vi "AutoVisionShoot.vi"(6 "Drive Params":T1={"Omni"=TRUE, "Low Gear"=TRUE}, 9 "Reset?":bool, 11 "Array":dbl[](array[numeric]) format="%0.3f") -> (3 "isFinished":bool)   [LabVIEW 2013]
uses:
  Shooter/Shooter Command.ctl
  Robot Global Data.vi
  Shooter/Shooter Manual Control.ctl
  Drivetrain/DT Mode.ctl
  Drivetrain/Drivetrain Control.ctl
  AutoDriveParams.ctl
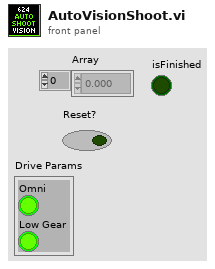
[diagram p1: front panel]
types:
  T1 = typedef "AutoDriveParams.ctl" = cluster{"Omni":bool, "Low Gear":bool}
  T2 = typedef "DT Mode.ctl" = enum16{"Manual", "Ball Steer", "Gyro Steer", "Goal Steer", "Catch Steer", "Selfcatch", "Ball Drive", "Distance Drive"}
  T3 = typedef "Drivetrain Control.ctl" = cluster{"axis 1 (x)":dbl, "axis 2 (y)":dbl, "Mode":T2, "heading target":dbl, "steer axis":dbl, "omni?":bool, "Low Gear?":bool, "distance target":cluster{"x":dbl, "y":dbl}, "PID Params":cluster{"X Dist":cluster{"PID gains":cluster{"proportional gain (Kc)":dbl, "integral time (Ti, min)":dbl, "derivative time (Td, min)":dbl}, "output range":cluster{"output high":dbl, "output low":dbl}}, "Y Dist":cluster{"PID gains":cluster{"proportional gain (Kc)":dbl, "integral time (Ti, min)":dbl, "derivative time (Td, min)":dbl}, "output range":cluster{"output high":dbl, "output low":dbl}}}, "Coast":bool}
  T4 = typedef "Shooter Manual Control.ctl" = cluster{"Command":T5, "Offset":dbl, "Trigger":bool, "Add":bool, "Release":bool, "Reset":bool, "Target Pressure":dbl, "Punch":bool, "AutoPunch":bool}
  T5 = typedef "Shooter Command.ctl" = enum16{"None", "Warmup", "Shoot", "Line Shoot"}
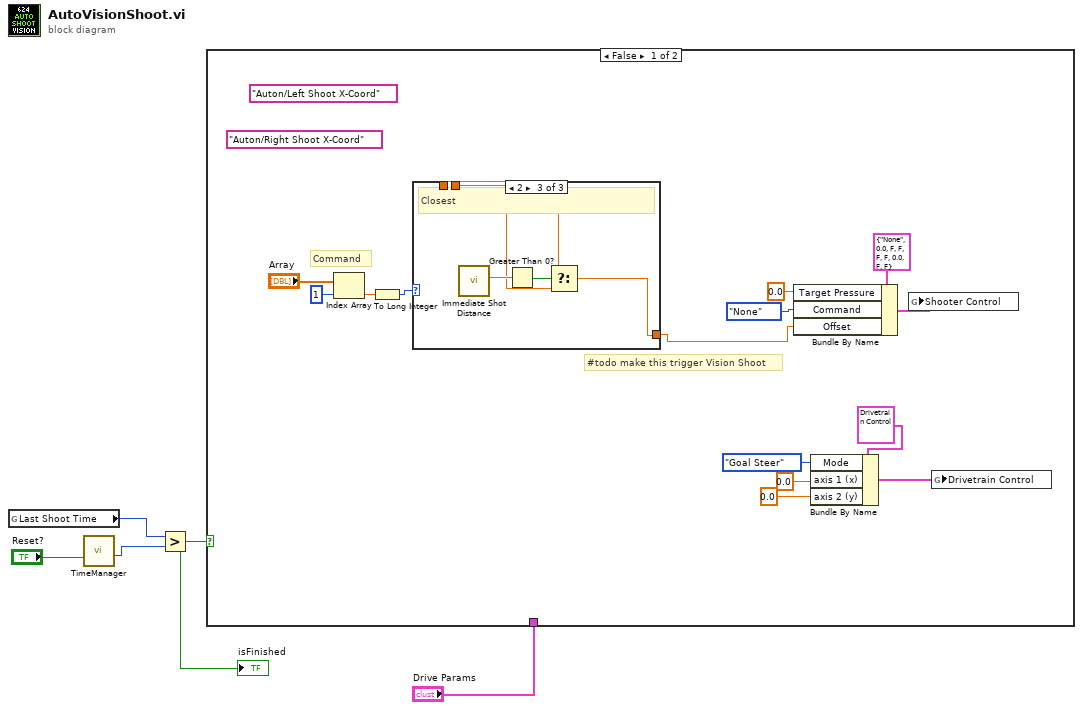
[diagram p0: block diagram]
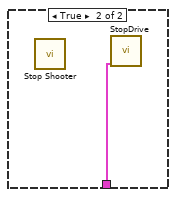
[diagram p4: hidden frame]
diagram:
  n1 = global read "Robot Global Data.vi" "Last Shoot Time"() -> (w4:u32)
  n2 = call "TimeManager.vi"("Reset?"="Reset?") -> ("Start Time"=w3:u32)  [unwired: 9 in, 1 out]
  n3 = Greater?(x=w4, y=w3) -> (0:w2:bool)
  "isFinished" <- w2
  n4 = case shown="False" w2 {
    tunnel: "Drive Params" -> [_ w31]
    frame False {
      w14 = "Auton/Left Shoot X-Coord" ("Name")
      w15 = "Auton/Right Shoot X-Coord" ("Name")
      # "#todo make this trigger Vision Shoot"
      # "Command"
      n5 = Index Array(array="Array", index=1) -> (element=w18:dbl)
      n6 = To Long Integer(number=w18) -> (32bit integer=w17:i32)
      n7 = case shown="2" w17 {
        tunnel: [w24 _ w28] -> w13
        tunnel: [_ w25 w27] -> w12
        tunnel: [w24 w25 w26] -> w11
        frame 0, Default {
          # "Left"
        }
        frame 1 {
          # "Right"
        }
        frame 2 {
          # "Closest"
          n8 = call "Immediate Shot Distance.vi"() -> ("Aimpoint X"=w30:dbl)  [unwired: 9 in, 2 out]
          n9 = Greater Than 0?(x=w30) -> (x > 0?=w29:bool)
          n10 = Select(t=w28, s=w29, f=w27) -> (s? t:f=w26:dbl)
        }
      }
      n11 = Bundle By Name(cluster=T4 {"Command"=enum."None", "Offset"=0.0, "Trigger"=FALSE, "Add"=FALSE, "Release"=FALSE, "Reset"=FALSE, "Target Pressure"=0.0, "Punch"=FALSE, "AutoPunch"=FALSE} ("Shooter Manual Control"), "Target Pressure"=0.0, "Command"=Shooter_Command."None" ("Enum"), "Offset"=w11) -> (w20:T4)
      n12 = Bundle By Name(cluster=T3 {"axis 1 (x)"=0.0, "axis 2 (y)"=0.0, "Mode"=enum."Manual", "heading target"=0.0, "steer axis"=0.0, "omni?"=FALSE, "Low Gear?"=FALSE, "distance target"={"x"=0.0, "y"=0.0}, "PID Params"={"X Dist"={"PID gains"={"proportional gain (Kc)"=1.0, "integral time (Ti, min)"=0.0, "derivative time (Td, min)"=0.0}, "output range"={"output high"=1.0, "output low"=-1.0}}, "Y Dist"={"PID gains"={"proportional gain (Kc)"=1.0, "integral time (Ti, min)"=0.0, "derivative time (Td, min)"=0.0}, "output range"={"output high"=1.0, "output low"=-1.0}}}, "Coast"=FALSE} ("Drivetrain Control"), "Mode"=DT_Mode."Goal Steer", "axis 1 (x)"=0.0, "axis 2 (y)"=0.0) -> (w10:T3)
      n13 = global write "Robot Global Data.vi" "Shooter Control"(w20) -> ()
      n14 = global write "Robot Global Data.vi" "Drivetrain Control"(w10) -> ()
    }
    frame True {
      n15 = call "Stop Shooter.vi"() -> ()  [unwired: 12 in]
      n16 = call "StopDrive.vi"("Drive Params"=w31) -> ()  [unwired: 11 in]
    }
  }
